vi "氨氮禁用写入 4.vi"(4 "error in (no error)":errorcluster caption="错误输入（无错误）", 5 "Value":T3(ring) caption="值", 6 "Container State":T2 caption="容器状态", 7 "Display State In":T1 caption="显示状态输入") -> (0 "error out":errorcluster caption="错误输出", 3 "Display State Out":T1 caption="显示状态输出")   [LabVIEW 2016, in "运维调试菜单.xctl"]
uses:
  <vilib>/_xctls/Container State.ctl
  <vilib>/_xctls/XControlSupport.lvlib
panel:
  # "将以下值显示控件替换为所需类型的显示控件。\n不要从连线板中删除该显示控件或其它显示控件。\n不要更改连线板模式。\n值显示控件应始终位于连线板输出端自顶部起第三个接线端。"
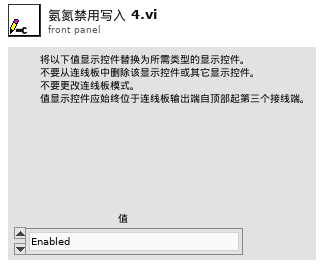
[diagram p1: front panel]
types:
  T1 = typedef "运维调试菜单.xctl/状态 1.ctl" = cluster{"采配水禁用":enum16{"Enabled", "Disabled", "Disabled and Grayed Out"}, "CODMn禁用":enum16{"Enabled", "Disabled", "Disabled and Grayed Out"}, "CODcr禁用":enum16{"Enabled", "Disabled", "Disabled and Grayed Out"}, "氨氮禁用":enum16{"Enabled", "Disabled", "Disabled and Grayed Out"}, "总磷总氮禁用":enum16{"Enabled", "Disabled", "Disabled and Grayed Out"}, "质控单元禁用":enum16{"Enabled", "Disabled", "Disabled and Grayed Out"}, "流量计禁用":enum16{"Enabled", "Disabled", "Disabled and Grayed Out"}, "电源管理禁用":enum16{"Enabled", "Disabled", "Disabled and Grayed Out"}, "其他禁用":enum16{"Enabled", "Disabled", "Disabled and Grayed Out"}, "多参数禁用":enum16{"Enabled", "Disabled", "Disabled and Grayed Out"}, "超标留样禁用":enum16{"Enabled", "Disabled", "Disabled and Grayed Out"}, "其他禁用":enum16{"Enabled", "Disabled", "Disabled and Grayed Out"}}
  T2 = typedef "XControlSupport.lvlib/Container State.ctl" = cluster{"Indicator?":bool, "Run Mode?":bool, " Refnum":refnum<vi>}
  T3 = enum16{"Enabled", "Disabled", "Disabled and Grayed Out"}
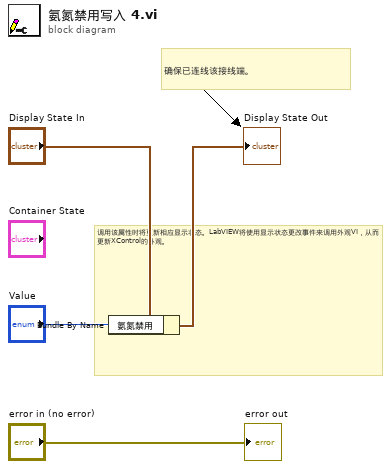
[diagram p0: block diagram]
diagram:
  # "确保已连线该接线端。"
  # "调用该属性时将更新相应显示状态。LabVIEW将使用显示状态更改事件来调用外观VI，从而更新XControl的外观。"
  n1 = Bundle By Name(cluster="Display State In", "氨氮禁用"="Value") -> (→"Display State Out":T1)
  "error out" <- "error in (no error)"
